vi "Attenuator Initialize Test VNA.vi"(0 "Instrument Record":T10, 5 "Parent VI Refnum":refnum<vi>, 7 "Timing Metrics In":string, 9 "Test Parameters In":T11={"Stimulus"={"ATT Stimulus"={"Normalize"=TRUE, "Value (dB)"=0.0}, "VNA Stimulus"={"Use Instrument Settings"=FALSE, "Blank Frequencies"=FALSE, "Sweep Type"=enum."Linear", "Sweep"={"Fstart"=500.0, "Fstop"=1500.0, "Units"=enum."MHz", "Points"=201}, "Power (dBm)"=999.0, "IFBW (Hz)"=-1.0, "Sweep Time (s)"=-1.0, "Calibration"={"State"=FALSE, "String"=""}}}, "Measurement"={"Step (dB)"=enum."0.25", "Start (dB)"=0.0, "Stop (dB)"=31.75}, "Limit"={"Maximum Error"=0.3}, "Normalization"={"Normalized?"=FALSE, "Normalization Values (dB)"=[]}} {"Stimulus"."VNA Stimulus"."Sweep Time (s)" format="%.3g"}, 11 "error in (no error)":errorcluster, 12 "Miscellaneous Parameters":T1) -> (4 "Instrument ID":string, 6 "Next Action":string, 8 "Timing Metrics Out":string, 10 "Test Parameters Out":T11={"Stimulus"={"ATT Stimulus"={"Normalize"=TRUE, "Value (dB)"=0.0}, "VNA Stimulus"={"Use Instrument Settings"=FALSE, "Blank Frequencies"=FALSE, "Sweep Type"=enum."Linear", "Sweep"={"Fstart"=500.0, "Fstop"=1500.0, "Units"=enum."MHz", "Points"=201}, "Power (dBm)"=999.0, "IFBW (Hz)"=-1.0, "Sweep Time (s)"=-1.0, "Calibration"={"State"=FALSE, "String"=""}}}, "Measurement"={"Step (dB)"=enum."0.25", "Start (dB)"=0.0, "Stop (dB)"=31.75}, "Limit"={"Maximum Error"=0.3}, "Normalization"={"Normalized?"=FALSE, "Normalization Values (dB)"=[]}} {"Stimulus"."VNA Stimulus"."Sweep Time (s)" format="%.3g"}, 14 "Driver Ref":T6, 15 "error out":errorcluster {"code" format="%.0x"})   [LabVIEW 2011]
uses:
  TypeDefs/Attenuator Test Parameters.ctl
  TypeDefs/Attenuator Stimulus Parameters.ctl
  TypeDefs/Attenuator ATT Stimulus.ctl
  TypeDefs/Attenuator VNA Stimulus.ctl
  S Parameter/TypeDefs/SP Frequency Units.ctl
  TypeDefs/Attenuator VNA Calibration State.ctl
  TypeDefs/Attenuator Measurement Cluster.ctl
  TypeDefs/Attenuator Limit.ctl
  TypeDefs/Attenuator Calibration State.ctl
  server/database/Stations/Instruments/Instrument Record.ctl
  TypeDefs/Attenuator Driver Refs.ctl
  drivers/ATT/ATT Driver Ref.ctl
  drivers/VNA/VNA Driver Ref.ctl
  drivers/SNA/SNA Driver Ref.ctl
  TypeDefs/Attenuator Parameter to Measure.ctl
  S Parameter/TypeDefs/SP Parameter.ctl
  S Parameter/TypeDefs/SP Measurement Format.ctl
  S Parameter/TypeDefs/SP Miscellaneous Parameters.ctl
  drivers/VNA/VNA Command.ctl
  drivers/SNA/SNA Command.ctl
panel:
  out "Parameters to Measure":T2[](array[typedef]) {"Channel" min=1 max=99 step=1; "Parameter"."Stimulus Port" min=1 step=1; "Parameter"."Response Port" min=1 step=1}
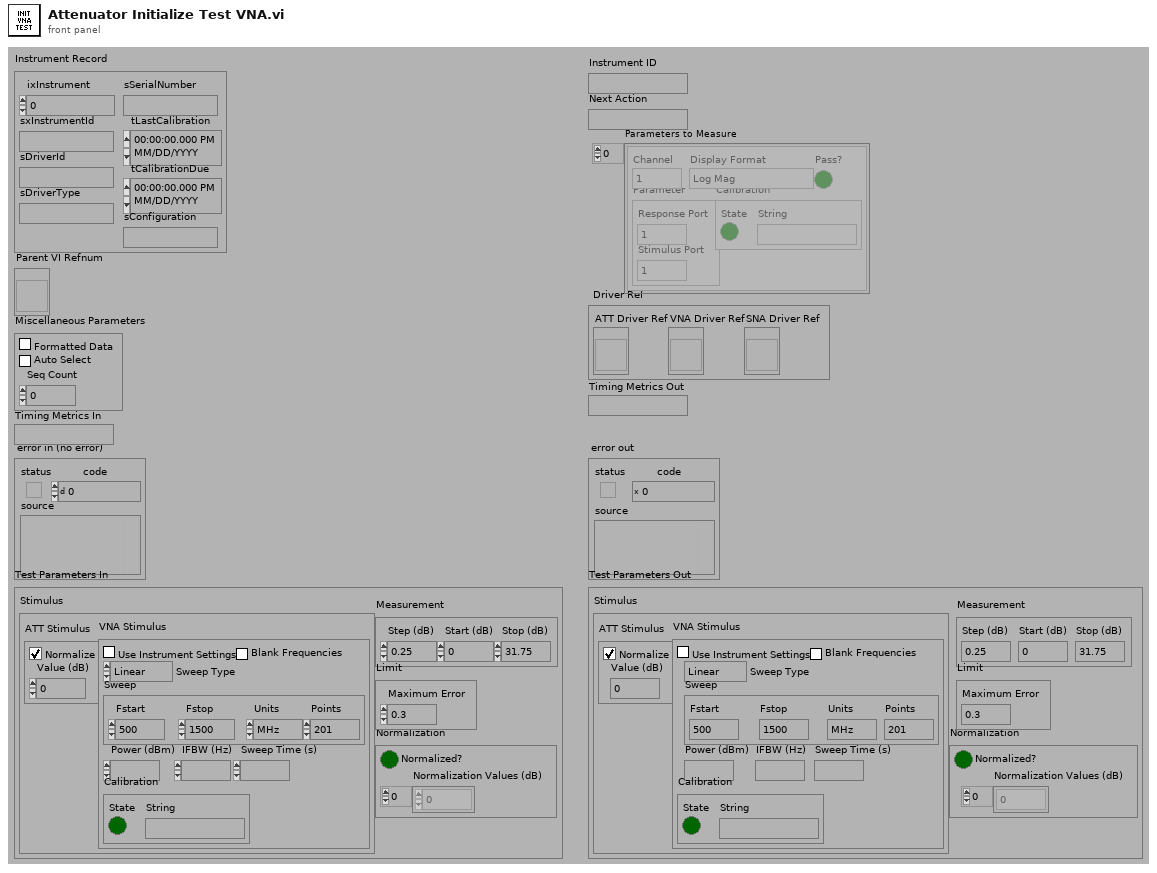
[diagram p1: front panel]
types:
  T1 = typedef "SP Miscellaneous Parameters.ctl" = cluster{"Formatted Data":bool, "Auto Select":bool, "Seq Count":u32}
  T2 = typedef "Attenuator Parameter to Measure.ctl" = cluster{"Channel":i8, "Parameter":T3, "Calibration":T4, "Display Format":T5, "Pass?":bool}
  T3 = typedef "SP Parameter.ctl" = cluster{"Stimulus Port":i8, "Response Port":i8}
  T4 = typedef "Attenuator VNA Calibration State.ctl" = cluster{"State":bool, "String":string}
  T5 = typedef "SP Measurement Format.ctl" = enum32{"Log Mag", "Phase", "Delay", "Smith (R+jX)", "Polar (Re/Im)", "Linear Mag", "SWR", "Real", "Imaginary", "Smith (Lin/Phase)", "Smith (Log/Phase)", "Smith (Real/Imag)", "Smith (G+jB)", "Polar (Lin/Phase)", "Polar (Log/Phase)", "Expanded Phase", "Positive Phase", "Inverted Smith", "Unwrapped Phase", "Power Out", "Power In", "Linear Mag/Phase", "Log Mag/Phase", "Real/Imaginary"}
  T6 = typedef "Attenuator Driver Refs.ctl" = cluster{"ATT Driver Ref":T7, "VNA Driver Ref":T8, "SNA Driver Ref":T9}
  T7 = typedef "ATT Driver Ref.ctl" = refnum<vi>
  T8 = typedef "VNA Driver Ref.ctl" = refnum<vi>
  T9 = typedef "SNA Driver Ref.ctl" = refnum<vi>
  T10 = typedef "Instrument Record.ctl" = cluster{"ixInstrument":i32, "sxInstrumentId":string, "sDriverId":string, "sDriverType":string, "sSerialNumber":string, "tLastCalibration":timestamp, "tCalibrationDue":timestamp, "sConfiguration":string}
  T11 = typedef "Attenuator Test Parameters.ctl" = cluster{"Stimulus":T12, "Measurement":T16, "Limit":T17, "Normalization":T18}
  T12 = typedef "Attenuator Stimulus Parameters.ctl" = cluster{"ATT Stimulus":T13, "VNA Stimulus":T14}
  T13 = typedef "Attenuator ATT Stimulus.ctl" = cluster{"Normalize":bool, "Value (dB)":dbl}
  T14 = typedef "Attenuator VNA Stimulus.ctl" = cluster{"Use Instrument Settings":bool, "Blank Frequencies":bool, "Sweep Type":enum32{"Linear", "Logarithmic", "List", "Power", "CW"}, "Sweep":cluster{"Fstart":dbl, "Fstop":dbl, "Units":T15, "Points":i32}, "Power (dBm)":dbl, "IFBW (Hz)":dbl, "Sweep Time (s)":dbl, "Calibration":T4}
  T15 = typedef "SP Frequency Units.ctl" = enum16{"Hz", "kHz", "MHz", "GHz", "Points"}
  T16 = typedef "Attenuator Measurement Cluster.ctl" = cluster{"Step (dB)":enum16{"0.25", "0.50", "1.00"}, "Start (dB)":dbl, "Stop (dB)":dbl}
  T17 = typedef "Attenuator Limit.ctl" = cluster{"Maximum Error":dbl}
  T18 = typedef "Attenuator Calibration State.ctl" = cluster{"Normalized?":bool, "Normalization Values (dB)":dbl[]}
  T19 = typedef "VNA Command.ctl" = enum16{"LOAD", "INITIALIZE", "PRESET", "GET STIMULUS", "SET STIMULUS", "GET CALIBRATION", "CALIBRATE", "RESTORE", "MEASURE", "RELEASE", "UNLOAD", "CONFIRM", "SORT"}
  T20 = typedef "SNA Command.ctl" = enum16{"LOAD", "INITIALIZE", "PRESET", "GET STIMULUS", "SET STIMULUS", "GET CALIBRATION", "CALIBRATE", "RESTORE", "MEASURE", "RELEASE", "UNLOAD", "CONFIRM", "SORT"}
  T21 = typedef "SP Parameter to Measure.ctl" = cluster{"Channel":i8, "Parameter":T3, "Calibration":T22, "Display Format":T5, "Pass?":bool}
  T22 = typedef "SP Calibration State.ctl" = cluster{"State":bool, "String":string}
  T23 = enum16{"None", "Calibrate", "Restore", "Ignore", "Abort"}
  T24 = typedef "Attenuator Dialog Response.ctl" = enum16{"None", "Calibrate", "Restore", "Ignore", "Abort", "Abort All"}
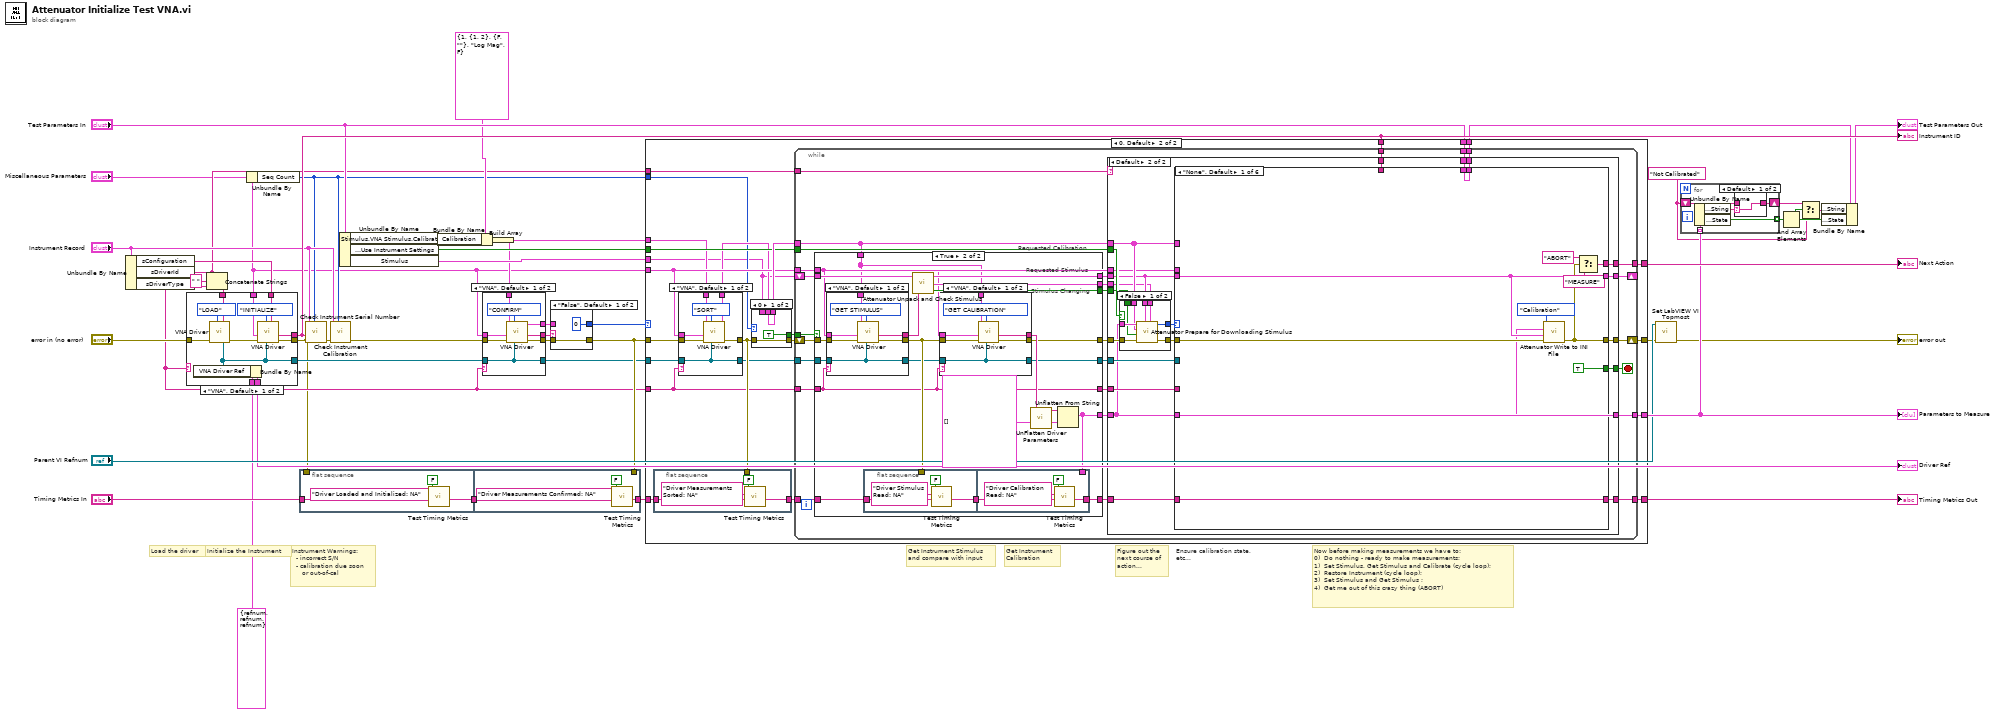
[diagram p0: block diagram]
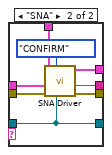
[diagram p3: hidden frame]
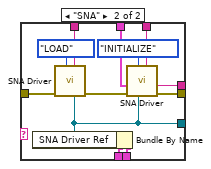
[diagram p4: hidden frame]
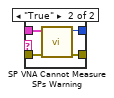
[diagram p5: hidden frame]
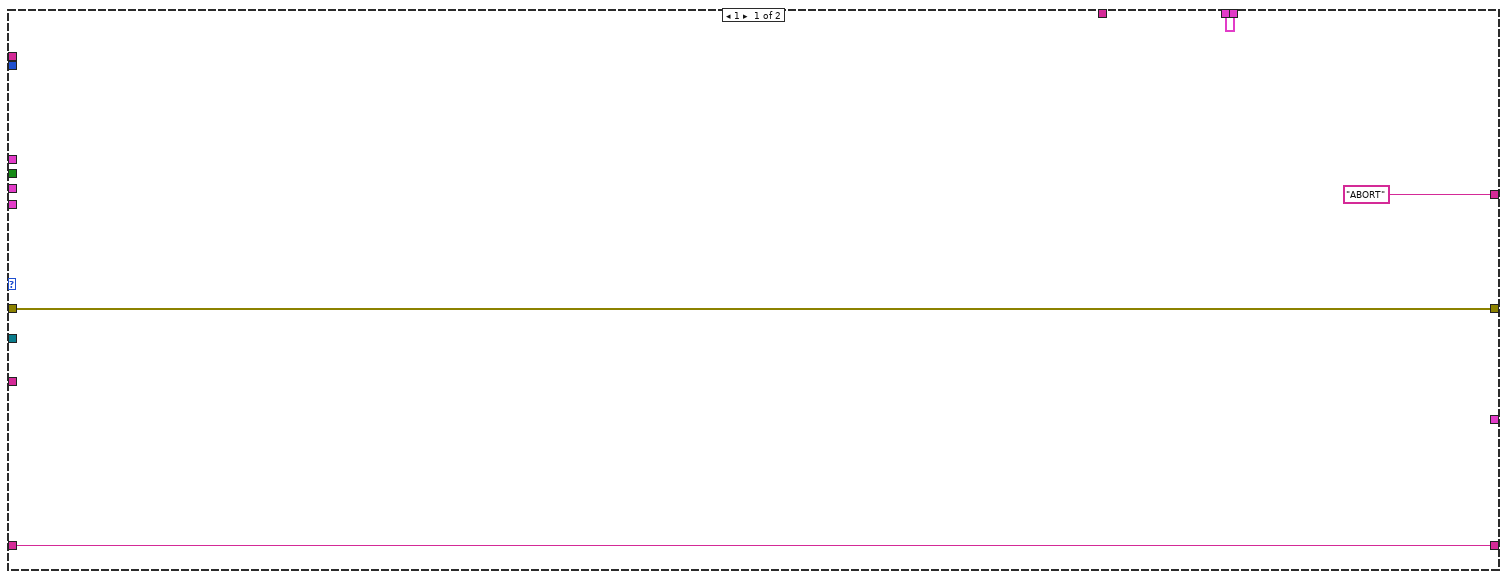
[diagram p6: hidden frame]
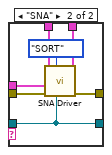
[diagram p7: hidden frame]
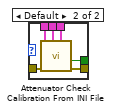
[diagram p8: hidden frame]
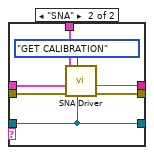
[diagram p10: hidden frame]
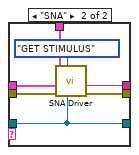
[diagram p11: hidden frame]
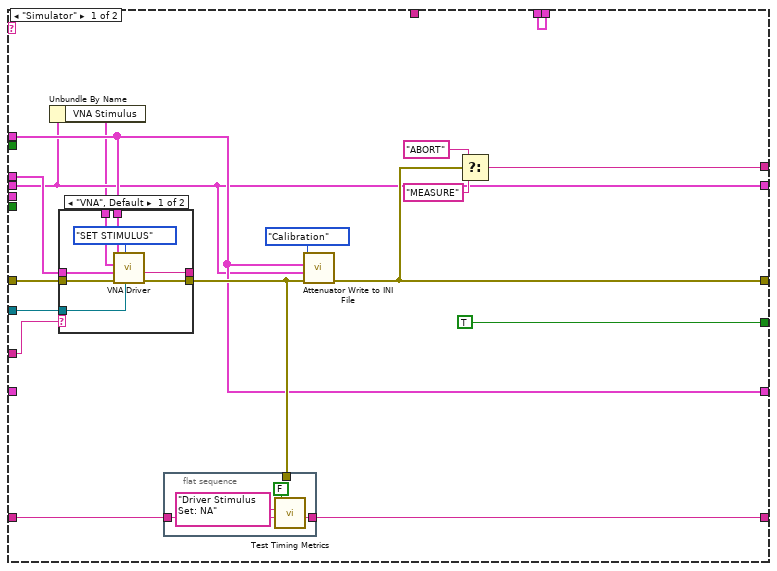
[diagram p12: hidden frame]
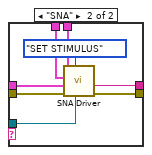
[diagram p13: hidden frame]
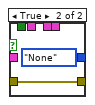
[diagram p14: hidden frame]
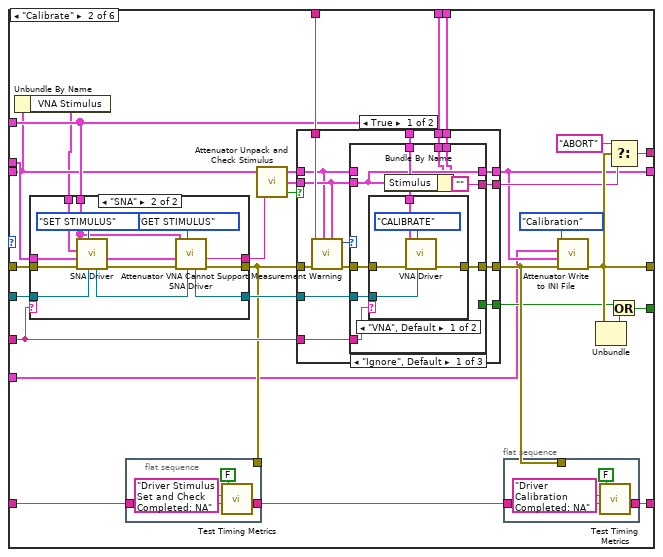
[diagram p15: hidden frame]
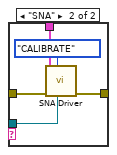
[diagram p16: hidden frame]
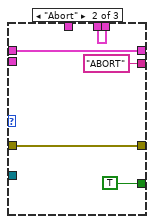
[diagram p17: hidden frame]
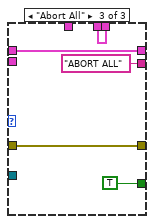
[diagram p18: hidden frame]
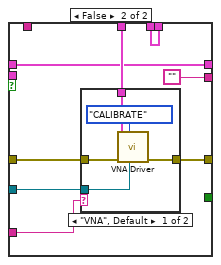
[diagram p19: hidden frame]
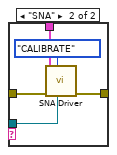
[diagram p20: hidden frame]
diagram:
  w5 = "Not Calibrated"
  # "Now before making measurements we have to:\n0)  Do nothing - ready to make measurements;\n1)  Set Stimulus, Get Stimulus and Calibrate (cycle loop);\n2)  Restore Instrument (cycle loop);\n3)  Set Stimulus and Get Stimulus ;\n4)  Get me out of this crazy thing (ABORT)"
  # "Figure out the\nnext course of\naction..."
  # "Get Instrument\nCalibration"
  # "Instrument Warnings:\n  - incorrect S/N\n  - calibration due soon\n     or out-of-cal"
  # "Get Instrument Stimulus\nand compare with input"
  # "Initialize the Instrument"
  # "Load the driver"
  n1 = Unbundle By Name("Instrument Record") -> ("sConfiguration"=w23:string, "sDriverId"=w22:string, "sDriverType"=w14:string)
  n2 = Concatenate Strings(w22, " " ("string"), w14) -> (w24:string)
  n3 = case shown="\"VNA\", Default" w14 {
    tunnel: "error in (no error)" -> [w55 w67]
    tunnel: [w54 w66] -> w45
    tunnel: w24 -> [w53 w65]
    tunnel: w23 -> [w52 w64]
    tunnel: T6 {"ATT Driver Ref"=refnum, "VNA Driver Ref"=refnum, "SNA Driver Ref"=refnum} ("Driver Ref") -> [w51 w63]
    tunnel: [w50 w62] -> w37
    tunnel: [w48 w58] -> w13
    tunnel: [w47 w60] -> w11
    tunnel: "Miscellaneous Parameters" -> [w46 w59]
    frame "VNA", Default {
      n4 = call "VNA Driver.vi"("VNA Driver or\nVNA Configuration (\"\")"=w53, "VNA Command"=VNA_Command."LOAD", "error in (no error)"=w55) -> ("error out"=w49:errorcluster, "dup Drv Refnum"=w48:T8)  [unwired: 4 in, 3 out]
      n5 = Bundle By Name(cluster=w51, "VNA Driver Ref"=w48) -> (w50:T6)
      n6 = call "VNA Driver.vi"("VNA Driver or\nVNA Configuration (\"\")"=w52, "Drv Refnum"=w48, "VNA Command"=VNA_Command."INITIALIZE", "error in (no error)"=w49, "Miscellaneous Parameters"=w46) -> ("error out"=w47:errorcluster, "VNA Flat Output"=w54:string)  [unwired: 2 in, 3 out]
    }
    frame "SNA" {
      n7 = call "SNA Driver.vi"("SNA Driver or\nSNA Configuration (\"\")"=w65, "SNA Command"=SNA_Command."LOAD", "error in (no error)"=w67) -> ("error out"=w61:errorcluster, "dup Drv Refnum"=w58:T9)  [unwired: 4 in, 3 out]
      n8 = Bundle By Name(cluster=w63, "SNA Driver Ref"=w58) -> (w62:T6)
      n9 = call "SNA Driver.vi"("SNA Driver or\nSNA Configuration (\"\")"=w64, "Drv Refnum"=w58, "SNA Command"=SNA_Command."INITIALIZE", "error in (no error)"=w61, "Miscellaneous Parameters"=w59) -> ("error out"=w60:errorcluster, "SNA Flat Output"=w66:string)  [unwired: 2 in, 3 out]
    }
  }
  "Instrument ID" <- w45
  "Driver Ref" <- w37
  n10 = Unbundle By Name("Miscellaneous Parameters") -> ("Seq Count"=w2:u32)
  n11 = flat-sequence {
    tunnel: [w71] -> w33
    tunnel: w11 -> [_]
    tunnel: "Timing Metrics In" -> [w70]
    tunnel: w33 -> [w75]
    tunnel: w16 -> [_]
    tunnel: [w74] -> w15
    frame #0 {
      n12 = call "Test Timing Metrics.vi"("Start?"=FALSE, "Timing Metrics In"=w70, "Message"="Driver Loaded and Initialized: NA") -> ("Timing Metrics Out"=w71:string)  [unwired: 6 out]
    }
    frame #1 {
      n13 = call "Test Timing Metrics.vi"("Start?"=FALSE, "Timing Metrics In"=w75, "Message"="Driver Measurements Confirmed: NA") -> ("Timing Metrics Out"=w74:string)  [unwired: 6 out]
    }
  }
  n14 = call "Check Instrument Serial Number.vi"("Seq Count"=w2, "error in (no error)"=w11, "Instrument IDN String (\"\")"=w45, "Instrument Record"="Instrument Record") -> ("error out"=w31:errorcluster)  [unwired: 7 out]
  n15 = call "Check Instrument Calibration.vi"("Seq Count"=w2, "error in (no error)"=w31, "Instrument Record"="Instrument Record") -> ("error out"=w21:errorcluster)  [unwired: 8 out]
  n16 = Unbundle By Name("Test Parameters In") -> ("Stimulus.VNA Stimulus.Calibration"=w28:T4, "Stimulus.VNA Stimulus.Use Instrument Settings"=w26:bool, "Stimulus"=w27:T12)
  n17 = Bundle By Name(cluster=T2 {"Channel"=1, "Parameter"={"Stimulus Port"=1, "Response Port"=2}, "Calibration"={"State"=FALSE, "String"=""}, "Display Format"=enum."Log Mag", "Pass?"=FALSE} ("Parameter to Measure"), "Calibration"=w28) -> (w4:T2)
  n18 = Build Array(w4) -> (w3:T2[])
  n19 = case shown="\"VNA\", Default" w14 {
    tunnel: w21 -> [w84 w92]
    tunnel: "Miscellaneous Parameters" -> [w83 w91]
    tunnel: [w82 w90] -> w20
    tunnel: [w81 w89] -> w19
    tunnel: w3 -> [w80 w88]
    tunnel: [w79 w87] -> w17
    tunnel: w13 -> [w78 w86]
    tunnel: [w78 w86] -> w12
    frame "VNA", Default {
      n20 = call "VNA Driver.vi"("Drv Refnum"=w78, "VNA Command"=VNA_Command."CONFIRM", "error in (no error)"=w84, "Miscellaneous Parameters"=w83, "Parameters to Measure"=w80) -> ("error out"=w79:errorcluster, "VNA Flat Output"=w82:string, "Parameters Measured"=w81:T21[])  [unwired: 2 in, 2 out]
    }
    frame "SNA" {
      n21 = call "SNA Driver.vi"("Drv Refnum"=w86, "SNA Command"=SNA_Command."CONFIRM", "error in (no error)"=w92, "Miscellaneous Parameters"=w91, "Parameters to Measure"=w88) -> ("error out"=w87:errorcluster, "SNA Flat Output"=w90:string, "Parameters Measured"=w89:T21[])  [unwired: 2 in, 2 out]
    }
  }
  n22 = case shown="\"False\", Default" w20 {
    tunnel: w17 -> [w95 w99]
    tunnel: [w95 w98] -> w16
    tunnel: w19 -> [_ w97]
    tunnel: [0 ("Choice") w96] -> w18
    frame "False", Default {
    }
    frame "True" {
      n23 = call "SP VNA Cannot Measure SPs Warning.vi"("error in (no error)"=w99, "Removed Parameters"=w97) -> ("error out"=w98:errorcluster, "Choice"=w96:i32)  [unwired: 8 out]
    }
  }
  n24 = case shown="0, Default" w18 {
    tunnel: ["ABORT" w127] -> w43
    tunnel: [_ w124] -> w42
    tunnel: [w103 w123] -> w30
    tunnel: w27 -> [_ w104]
    tunnel: w26 -> [_ w121]
    tunnel: w22 -> [_ w120]
    tunnel: w16 -> [w103 w115]
    tunnel: "Miscellaneous Parameters" -> [_ w114]
    tunnel: w3 -> [_ w113]
    tunnel: w15 -> [w101 w119]
    tunnel: [w101 w117] -> w35
    tunnel: w14 -> [_ w109]
    tunnel: w12 -> [_ w111]
    tunnel: w45 -> [_ w108]
    tunnel: "Test Parameters In" -> [w100 w107]
    tunnel: [w100 w106] -> w9
    tunnel: w2 -> [_ w105]
    frame 1 {
    }
    frame 0, Default {
      n25 = flat-sequence {
        tunnel: w119 -> [w143]
        tunnel: [w142] -> w118
        tunnel: w116 -> [_]
        frame #0 {
          n26 = call "Test Timing Metrics.vi"("Start?"=FALSE, "Timing Metrics In"=w143, "Message"="Driver Measurements Sorted: NA") -> ("Timing Metrics Out"=w142:string)  [unwired: 6 out]
        }
      }
      n27 = case shown="\"VNA\", Default" w109 {
        tunnel: w115 -> [w133 w140]
        tunnel: w114 -> [w132 w139]
        tunnel: w113 -> [w131 w138]
        tunnel: [w130 w137] -> w116
        tunnel: [w129 w136] -> w112
        tunnel: w111 -> [w128 w135]
        tunnel: [w128 w135] -> w110
        frame "VNA", Default {
          n28 = call "VNA Driver.vi"("Drv Refnum"=w128, "VNA Command"=VNA_Command."SORT", "error in (no error)"=w133, "Miscellaneous Parameters"=w132, "Parameters to Measure"=w131) -> ("error out"=w130:errorcluster, "Parameters Measured"=w129:T21[])  [unwired: 2 in, 3 out]
        }
        frame "SNA" {
          n29 = call "SNA Driver.vi"("Drv Refnum"=w135, "SNA Command"=SNA_Command."SORT", "error in (no error)"=w140, "Miscellaneous Parameters"=w139, "Parameters to Measure"=w138) -> ("error out"=w137:errorcluster, "Parameters Measured"=w136:T21[])  [unwired: 2 in, 3 out]
        }
      }
      n30 = case shown="0" w105 {
        tunnel: w116 -> [w148 w154]
        tunnel: [w148 w153] -> w126
        tunnel: [TRUE ("Check Instrument") w152] -> w125
        tunnel: w112 -> [w146 w151]
        tunnel: w104 -> [_ w150]
        tunnel: [w146 w149] -> w122
        frame 0 {
        }
        frame Default {
          n31 = call "Attenuator Check Calibration From INI File.vi"("Paramters to Measure"=w151, "error in (no error)"=w154, "Requested Stimulus"=w150) -> ("error out"=w153:errorcluster, "Check Instrument"=w152:bool, "Paramters to Measure Out"=w149:T2[])  [unwired: 5 in, 1 out]
        }
      }
      n32 = while "Ensure calibration state, etc..." {
        shift-right: [w180] -> w123
        shift-left: w126 -> [w169]
        tunnel: [w179] -> w127
        tunnel: [w177] -> w124
        tunnel: w120 -> [w176]
        tunnel: w122 -> [w155]
        tunnel: w125 -> [w170]
        tunnel: w121 -> [w168]
        tunnel: w114 -> [w166]
        tunnel: w118 -> [w165]
        tunnel: [w163] -> w117
        tunnel: w110 -> [w162]
        tunnel: w109 -> [w161]
        tunnel: w108 -> [w159]
        tunnel: w107 -> [w158]
        tunnel: [w157] -> w106
        shift-right: [w156] -> _
        shift-left: w104 -> [w171]
        stop <- w181 stop-if-true
        # "Requested Calibration"
        n33 = case shown="True" w170 {
          selector: w170 -> [w187 _]
          tunnel: [w182 w202] -> w178
          tunnel: [w188 w196] -> w175
          tunnel: [w187 w207] -> w174
          tunnel: [w186 w208] -> w173
          tunnel: w169 -> [w188 w200]
          tunnel: w171 -> [w186 w206]
          tunnel: [w184 w192] -> w172
          tunnel: [w186 w205] -> w167
          tunnel: w155 -> [w182 w191]
          tunnel: w166 -> [_ w195]
          tunnel: w165 -> [w185 w204]
          tunnel: [w185 w201] -> w164
          tunnel: w162 -> [w184 w199]
          tunnel: w161 -> [w183 w190]
          tunnel: [w183 w190] -> w160
          frame False {
            # "Don't check instrument.\nSettings are the same as last run.\nSave time."
          }
          frame True {
            # "Requested Stimulus"
            # "Stimulus Changing"
            n34 = case shown="\"VNA\", Default" w190 {
              tunnel: w200 -> [w230 w237]
              tunnel: w195 -> [w229 w236]
              tunnel: w191 -> [w228 w235]
              tunnel: [w227 w234] -> w194
              tunnel: w199 -> [w226 w233]
              tunnel: [w226 w233] -> w193
              tunnel: [w225 w232] -> w198
              frame "VNA", Default {
                n35 = call "VNA Driver.vi"("Drv Refnum"=w226, "VNA Command"=VNA_Command."GET STIMULUS", "error in (no error)"=w230, "Miscellaneous Parameters"=w229, "Parameters to Measure"=w228) -> ("error out"=w227:errorcluster, "VNA Flat Output"=w225:string)  [unwired: 2 in, 3 out]
              }
              frame "SNA" {
                n36 = call "SNA Driver.vi"("Drv Refnum"=w233, "SNA Command"=SNA_Command."GET STIMULUS", "error in (no error)"=w237, "Miscellaneous Parameters"=w236, "Parameters to Measure"=w235) -> ("error out"=w234:errorcluster, "SNA Flat Output"=w232:string)  [unwired: 2 in, 3 out]
              }
            }
            n37 = flat-sequence {
              tunnel: w204 -> [w239]
              tunnel: w194 -> [_]
              tunnel: [w238] -> w203
              tunnel: w203 -> [w243]
              tunnel: w202 -> [_]
              tunnel: [w242] -> w201
              frame #0 {
                n38 = call "Test Timing Metrics.vi"("Start?"=FALSE, "Timing Metrics In"=w239, "Message"="Driver Stimulus Read: NA") -> ("Timing Metrics Out"=w238:string)  [unwired: 6 out]
              }
              frame #1 {
                n39 = call "Test Timing Metrics.vi"("Start?"=FALSE, "Timing Metrics In"=w243, "Message"="Driver Calibration Read: NA") -> ("Timing Metrics Out"=w242:string)  [unwired: 6 out]
              }
            }
            n40 = call "Attenuator Unpack and Check Stimulus.vi"("Flat Stimulus"=w198, "Requested Stimulus In"=w206) -> ("Stimulus Changed?"=w207:bool, "Current Stimulus"=w205:T12, "Requested Stimulus Out"=w208:T12)  [unwired: 1 out]
            n41 = case shown="\"VNA\", Default" w190 {
              tunnel: w194 -> [w216 w223]
              tunnel: w195 -> [w215 w222]
              tunnel: w191 -> [w214 w221]
              tunnel: [w213 w220] -> w196
              tunnel: w193 -> [w212 w219]
              tunnel: [w212 w219] -> w192
              tunnel: [w211 w218] -> w197
              frame "VNA", Default {
                n42 = call "VNA Driver.vi"("Drv Refnum"=w212, "VNA Command"=VNA_Command."GET CALIBRATION", "error in (no error)"=w216, "Miscellaneous Parameters"=w215, "Parameters to Measure"=w214) -> ("error out"=w213:errorcluster, "VNA Flat Output"=w211:string)  [unwired: 2 in, 3 out]
              }
              frame "SNA" {
                n43 = call "SNA Driver.vi"("Drv Refnum"=w219, "SNA Command"=SNA_Command."GET CALIBRATION", "error in (no error)"=w223, "Miscellaneous Parameters"=w222, "Parameters to Measure"=w221) -> ("error out"=w220:errorcluster, "SNA Flat Output"=w218:string)  [unwired: 2 in, 3 out]
              }
            }
            n44 = call "UnFlatten Driver Parameters.vi"("Flattened Driver Parameters with Version (\"\")"=w197) -> ("Flat Driver Parameters"=w209:string)  [unwired: 1 in, 5 out]
            n45 = Unflatten From String(type=T2[] [] ("Parameters Measured"), binary string=w209) -> (value=w202:T2[])  [unwired: 1 in, 4 out]
          }
        }
        n46 = case shown="Default" w176 {
          tunnel: [TRUE w303] -> w181
          tunnel: [w258 w302] -> w180
          tunnel: [w260 w301] -> w179
          tunnel: w173 -> [w247 w294]
          tunnel: w172 -> [w251 w300]
          tunnel: w178 -> [_ w283]
          tunnel: [w248 w283] -> w177
          tunnel: w175 -> [w253 w299]
          tunnel: w155 -> [w248 w296]
          tunnel: w174 -> [_ w288]
          tunnel: w168 -> [_ w295]
          tunnel: w167 -> [_ w293]
          tunnel: w166 -> [w254 w292]
          tunnel: w164 -> [w255 w291]
          tunnel: [w256 w290] -> w163
          tunnel: w160 -> [w250 w289]
          tunnel: w159 -> [_ w287]
          tunnel: w158 -> [w249 w286]
          tunnel: [w249 w285] -> w157
          tunnel: [w247 w284] -> w156
          frame "Simulator" {
            n47 = Unbundle By Name(w247) -> ("VNA Stimulus"=w246:T14)
            n48 = case shown="\"VNA\", Default" w250 {
              tunnel: w253 -> [w270 w278]
              tunnel: w254 -> [w269 w277]
              tunnel: w248 -> [w268 w276]
              tunnel: [w267 w275] -> w252
              tunnel: w251 -> [w266 w274]
              tunnel: [w265 w273] -> _
              tunnel: w246 -> [w263 w271]
              frame "VNA", Default {
                n49 = call "VNA Driver.vi"("Drv Refnum"=w266, "VNA Command"=VNA_Command."SET STIMULUS", "error in (no error)"=w270, "Miscellaneous Parameters"=w269, "VNA Stimulus"=w263, "Parameters to Measure"=w268) -> ("error out"=w267:errorcluster, "VNA Flat Output"=w265:string)  [unwired: 1 in, 3 out]
              }
              frame "SNA" {
                n50 = call "SNA Driver.vi"("Drv Refnum"=w274, "SNA Command"=SNA_Command."SET STIMULUS", "error in (no error)"=w278, "Miscellaneous Parameters"=w277, "SNA Stimulus"=w271, "Parameters to Measure"=w276) -> ("error out"=w275:errorcluster, "SNA Flat Output"=w273:string)  [unwired: 1 in, 3 out]
              }
            }
            n51 = flat-sequence {
              tunnel: [w279] -> w256
              tunnel: w255 -> [w280]
              tunnel: w252 -> [_]
              frame #0 {
                n52 = call "Test Timing Metrics.vi"("Start?"=FALSE, "Timing Metrics In"=w280, "Message"="Driver Stimulus Set: NA") -> ("Timing Metrics Out"=w279:string)  [unwired: 6 out]
              }
            }
            n53 = call "Attenuator Write to INI File.vi"("error in (no error)"=w252, "Requested Stimulus"=w247, "Parameters to Measure"=w248, "Data to Write"=enum16{"Calibration", "Display", "De-Embed"}."Calibration") -> ("error out"=w258:errorcluster)  [unwired: 2 in, 5 out]
            n54 = Select(t="ABORT", s=w258, f="MEASURE") -> (s? t:f=w260:string)
          }
          frame Default {
            n55 = case shown="False" w295 {
              tunnel: w299 -> [w311 w313]
              tunnel: [w310 w313] -> w298
              tunnel: [w309 T23."None" ("Action")] -> w297
              tunnel: w283 -> [w308 _]
              tunnel: w288 -> [w307 _]
              tunnel: w296 -> [w306 _]
              tunnel: w294 -> [w305 _]
              tunnel: w293 -> [w304 _]
              frame False {
                n56 = call "Attenuator Prepare for Downloading Stimulus.vi"("Current Stimulus"=w304, "Requested Stimulus"=w305, "error in (no error)"=w311, "Stimulus Changing? (f)"=w307, "Parameters to Measure"=w306, "Currnet Parameters to Measure"=w308) -> ("error out"=w310:errorcluster, "Action"=w309:T24)  [unwired: 1 in, 3 out]
              }
              frame True {
              }
            }
            n57 = case shown="\"None\", Default" w297 {
              tunnel: w298 -> [w320 w349 w456 w490 w569 w577]
              tunnel: [w319 w352 w460 w501 w568 w576] -> w302
              tunnel: [TRUE w334 w461 TRUE TRUE TRUE] -> w303
              tunnel: [w322 w353 w462 w505 "ABORT" "ABORT ALL"] -> w301
              tunnel: w300 -> [_ w348 w454 w498 _ _]
              tunnel: w296 -> [_ w327 w449 w481 _ _]
              tunnel: w294 -> [w315 w326 w451 w480 w565 w573]
              tunnel: w292 -> [_ w347 _ w489 _ _]
              tunnel: w291 -> [w317 w342 w458 w497 w567 w575]
              tunnel: [w317 w350 w457 w496 w567 w575] -> w290
              tunnel: w289 -> [_ w344 w453 w491 _ _]
              tunnel: w287 -> [_ w339 _ w487 _ _]
              tunnel: w286 -> [w316 w331 w452 w485 w566 w574]
              tunnel: [w316 w330 w452 w484 w566 w574] -> w285
              tunnel: [w315 w329 w451 w483 w565 w573] -> w284
              tunnel: w283 -> [w314 w328 w450 w482 w564 w572]
              frame "None", Default {
                n58 = call "Attenuator Write to INI File.vi"("error in (no error)"=w320, "Requested Stimulus"=w315, "Parameters to Measure"=w314, "Data to Write"=enum16{"Calibration", "Display", "De-Embed"}."Calibration") -> ("error out"=w319:errorcluster)  [unwired: 2 in, 5 out]
                n59 = Select(t="ABORT", s=w319, f="MEASURE") -> (s? t:f=w322:string)
              }
              frame "Calibrate" {
                n60 = Unbundle By Name(w326) -> ("VNA Stimulus"=w325:T14)
                n61 = case shown="\"SNA\"" w344 {
                  tunnel: w349 -> [w432 w444]
                  tunnel: w347 -> [w431 w435]
                  tunnel: w327 -> [w424 w439]
                  tunnel: [w427 w440] -> w340
                  tunnel: w348 -> [w429 w438]
                  tunnel: [w423 w436] -> w345
                  tunnel: [w422 w434] -> w343
                  tunnel: w325 -> [w421 w433]
                  frame "VNA", Default {
                    n62 = call "VNA Driver.vi"("Drv Refnum"=w429, "VNA Command"=VNA_Command."SET STIMULUS", "error in (no error)"=w432, "Miscellaneous Parameters"=w431, "VNA Stimulus"=w421, "Parameters to Measure"=w424) -> ("error out"=w425:errorcluster, "dup Drv Refnum"=w428:T8)  [unwired: 1 in, 3 out]
                    n63 = call "VNA Driver.vi"("Drv Refnum"=w428, "VNA Command"=VNA_Command."GET STIMULUS", "error in (no error)"=w425, "Parameters to Measure"=w424) -> ("error out"=w427:errorcluster, "VNA Flat Output"=w422:string, "dup Drv Refnum"=w423:T8)  [unwired: 3 in, 2 out]
                  }
                  frame "SNA" {
                    n64 = call "SNA Driver.vi"("Drv Refnum"=w438, "SNA Command"=SNA_Command."SET STIMULUS", "error in (no error)"=w444, "Miscellaneous Parameters"=w435, "SNA Stimulus"=w433, "Parameters to Measure"=w439) -> ("error out"=w441:errorcluster, "dup Drv Refnum"=w437:T9)  [unwired: 1 in, 3 out]
                    n65 = call "SNA Driver.vi"("Drv Refnum"=w437, "SNA Command"=SNA_Command."GET STIMULUS", "error in (no error)"=w441, "Miscellaneous Parameters"=w435, "Parameters to Measure"=w439) -> ("error out"=w440:errorcluster, "SNA Flat Output"=w434:string, "dup Drv Refnum"=w436:T9)  [unwired: 2 in, 2 out]
                  }
                }
                n66 = flat-sequence {
                  tunnel: [w418] -> w341
                  tunnel: w342 -> [w417]
                  tunnel: w340 -> [_]
                  frame #0 {
                    n67 = call "Test Timing Metrics.vi"("Start?"=FALSE, "Timing Metrics In"=w417, "Message"="Driver Stimulus Set and Check Completed: NA") -> ("Timing Metrics Out"=w418:string)  [unwired: 6 out]
                  }
                }
                n68 = call "Attenuator Unpack and Check Stimulus.vi"("Flat Stimulus"=w343, "Requested Stimulus In"=w326) -> ("Stimulus Changed?"=w338:bool, "Current Stimulus"=w337:T12, "Requested Stimulus Out"=w336:T12)  [unwired: 1 out]
                n69 = case shown="True" w338 {
                  tunnel: [w369 w406] -> w346
                  tunnel: w345 -> [w368 w405]
                  tunnel: w327 -> [w367 w404]
                  tunnel: w344 -> [w366 w403]
                  tunnel: w340 -> [w364 w401]
                  tunnel: w339 -> [w363 _]
                  tunnel: w337 -> [w361 _]
                  tunnel: w336 -> [w360 w400]
                  tunnel: [w359 w400] -> w329
                  tunnel: [w358 ""] -> w335
                  tunnel: [w357 _] -> w332
                  tunnel: w331 -> [w356 w399]
                  tunnel: [w355 w399] -> w330
                  frame True {
                    n70 = call "Attenuator VNA Cannot Support Measurement Warning.vi"("Current Stimulus"=w361, "Requested Stimulus"=w360, "error in (no error)"=w364, "Instrument IDN String (\"\")"=w363) -> ("error out"=w365:errorcluster, "Choice"=w362:T24)  [unwired: 2 in, 4 out]
                    n71 = case shown="\"Ignore\", Default" w362 {
                      tunnel: [w378 w391 w396] -> w369
                      tunnel: w368 -> [w377 _ _]
                      tunnel: w367 -> [w376 _ _]
                      tunnel: w366 -> [w375 _ _]
                      tunnel: w365 -> [w374 w391 w396]
                      tunnel: w361 -> [w372 _ _]
                      tunnel: w360 -> [_ w393 w398]
                      tunnel: [w372 w393 w398] -> w359
                      tunnel: ["" "ABORT" "ABORT ALL"] -> w358
                      tunnel: [_ TRUE TRUE] -> w357
                      tunnel: w356 -> [w371 w389 w394]
                      tunnel: [w370 w389 w394] -> w355
                      frame "Ignore", Default {
                        n72 = case shown="\"VNA\", Default" w375 {
                          tunnel: w374 -> [w383 w388]
                          tunnel: w376 -> [w380 w386]
                          tunnel: [w379 w384] -> w378
                          tunnel: w377 -> [w381 w385]
                          frame "VNA", Default {
                            n73 = call "VNA Driver.vi"("Drv Refnum"=w381, "VNA Command"=VNA_Command."CALIBRATE", "error in (no error)"=w383, "Parameters to Measure"=w380) -> ("error out"=w379:errorcluster)  [unwired: 3 in, 4 out]
                          }
                          frame "SNA" {
                            n74 = call "SNA Driver.vi"("Drv Refnum"=w385, "SNA Command"=SNA_Command."CALIBRATE", "error in (no error)"=w388, "Parameters to Measure"=w386) -> ("error out"=w384:errorcluster)  [unwired: 3 in, 4 out]
                          }
                        }
                        n75 = Bundle By Name(cluster=w371, "Stimulus"=w372) -> (w370:T11)
                      }
                      frame "Abort" {
                      }
                      frame "Abort All" {
                      }
                    }
                  }
                  frame False {
                    n76 = case shown="\"VNA\", Default" w403 {
                      tunnel: w401 -> [w411 w416]
                      tunnel: w404 -> [w408 w414]
                      tunnel: [w407 w412] -> w406
                      tunnel: w405 -> [w409 w413]
                      frame "VNA", Default {
                        n77 = call "VNA Driver.vi"("Drv Refnum"=w409, "VNA Command"=VNA_Command."CALIBRATE", "error in (no error)"=w411, "Parameters to Measure"=w408) -> ("error out"=w407:errorcluster)  [unwired: 3 in, 4 out]
                      }
                      frame "SNA" {
                        n78 = call "SNA Driver.vi"("Drv Refnum"=w413, "SNA Command"=SNA_Command."CALIBRATE", "error in (no error)"=w416, "Parameters to Measure"=w414) -> ("error out"=w412:errorcluster)  [unwired: 3 in, 4 out]
                      }
                    }
                  }
                }
                n79 = flat-sequence {
                  tunnel: [w446] -> w350
                  tunnel: w341 -> [w445]
                  tunnel: w346 -> [_]
                  frame #0 {
                    n80 = call "Test Timing Metrics.vi"("Start?"=FALSE, "Timing Metrics In"=w445, "Message"="Driver Calibration Completed: NA") -> ("Timing Metrics Out"=w446:string)  [unwired: 6 out]
                  }
                }
                n81 = call "Attenuator Write to INI File.vi"("error in (no error)"=w346, "Requested Stimulus"=w329, "Parameters to Measure"=w328, "Data to Write"=enum16{"Calibration", "Display"}."Calibration") -> ("error out"=w352:errorcluster)  [unwired: 2 in, 5 out]
                n82 = Unbundle(w352) -> ("status"=w333:bool)  [unwired: 2 out]
                n83 = Select(t="ABORT", s=w352, f=w335) -> (s? t:f=w353:string)
                n84 = Or(x=w332, y=w333) -> (x .or. y?=w334:bool)
              }
              frame "Restore" {
                n85 = case shown="\"SNA\"" w453 {
                  tunnel: w456 -> [w469 w474]
                  tunnel: w449 -> [w468 w473]
                  tunnel: [w467 w472] -> w455
                  tunnel: w454 -> [w466 w471]
                  frame "VNA", Default {
                    n86 = call "VNA Driver.vi"("Drv Refnum"=w466, "VNA Command"=VNA_Command."RESTORE", "error in (no error)"=w469, "Parameters to Measure"=w468) -> ("error out"=w467:errorcluster)  [unwired: 3 in, 4 out]
                  }
                  frame "SNA" {
                    n87 = call "SNA Driver.vi"("Drv Refnum"=w471, "SNA Command"=SNA_Command."RESTORE", "error in (no error)"=w474, "Parameters to Measure"=w473) -> ("error out"=w472:errorcluster)  [unwired: 3 in, 4 out]
                  }
                }
                n88 = flat-sequence {
                  tunnel: w458 -> [w476]
                  tunnel: w455 -> [_]
                  tunnel: [w475] -> w457
                  frame #0 {
                    n89 = call "Test Timing Metrics.vi"("Start?"=FALSE, "Timing Metrics In"=w476, "Message"="Driver Calibration Restored: NA") -> ("Timing Metrics Out"=w475:string)  [unwired: 6 out]
                  }
                }
                n90 = call "Attenuator Write to INI File.vi"("error in (no error)"=w455, "Requested Stimulus"=w451, "Parameters to Measure"=w450, "Data to Write"=enum16{"Calibration", "Display", "De-Embed"}."Calibration") -> ("error out"=w460:errorcluster)  [unwired: 2 in, 5 out]
                n91 = Unbundle(w460) -> ("status"=w461:bool)  [unwired: 2 out]
                n92 = Select(t="ABORT", s=w460, f="") -> (s? t:f=w462:string)
              }
              frame "Ignore" {
                n93 = Unbundle By Name(w480) -> ("VNA Stimulus"=w479:T14)
                n94 = case shown="\"SNA\"" w491 {
                  tunnel: w490 -> [w551 w563]
                  tunnel: w489 -> [w550 w554]
                  tunnel: w481 -> [w543 w558]
                  tunnel: [w546 w559] -> w499
                  tunnel: w498 -> [w548 w557]
                  tunnel: [w542 w555] -> w488
                  tunnel: [w541 w553] -> w500
                  tunnel: w479 -> [w540 w552]
                  frame "VNA", Default {
                    n95 = call "VNA Driver.vi"("Drv Refnum"=w548, "VNA Command"=VNA_Command."SET STIMULUS", "error in (no error)"=w551, "Miscellaneous Parameters"=w550, "VNA Stimulus"=w540, "Parameters to Measure"=w543) -> ("error out"=w544:errorcluster, "dup Drv Refnum"=w547:T8)  [unwired: 1 in, 3 out]
                    n96 = call "VNA Driver.vi"("Drv Refnum"=w547, "VNA Command"=VNA_Command."GET STIMULUS", "error in (no error)"=w544, "Parameters to Measure"=w543) -> ("error out"=w546:errorcluster, "VNA Flat Output"=w541:string, "dup Drv Refnum"=w542:T8)  [unwired: 3 in, 2 out]
                  }
                  frame "SNA" {
                    n97 = call "SNA Driver.vi"("Drv Refnum"=w557, "SNA Command"=SNA_Command."SET STIMULUS", "error in (no error)"=w563, "Miscellaneous Parameters"=w554, "SNA Stimulus"=w552, "Parameters to Measure"=w558) -> ("error out"=w560:errorcluster, "dup Drv Refnum"=w556:T9)  [unwired: 1 in, 3 out]
                    n98 = call "SNA Driver.vi"("Drv Refnum"=w556, "SNA Command"=SNA_Command."GET STIMULUS", "error in (no error)"=w560, "Miscellaneous Parameters"=w554, "Parameters to Measure"=w558) -> ("error out"=w559:errorcluster, "SNA Flat Output"=w553:string, "dup Drv Refnum"=w555:T9)  [unwired: 2 in, 2 out]
                  }
                }
                n99 = flat-sequence {
                  tunnel: [w537] -> w496
                  tunnel: w497 -> [w536]
                  tunnel: w499 -> [_]
                  frame #0 {
                    n100 = call "Test Timing Metrics.vi"("Start?"=FALSE, "Timing Metrics In"=w536, "Message"="Driver Stimulus Set and Check Completed: NA") -> ("Timing Metrics Out"=w537:string)  [unwired: 6 out]
                  }
                }
                n101 = call "Attenuator Unpack and Check Stimulus.vi"("Flat Stimulus"=w500, "Requested Stimulus In"=w480) -> ("Stimulus Changed?"=w494:bool, "Current Stimulus"=w493:T12, "Requested Stimulus Out"=w492:T12)  [unwired: 1 out]
                n102 = case shown="False" w494 {
                  tunnel: [w518 w534] -> w495
                  tunnel: w488 -> [w517 _]
                  tunnel: w491 -> [w516 _]
                  tunnel: w499 -> [w514 w534]
                  tunnel: w487 -> [w513 _]
                  tunnel: w493 -> [w511 _]
                  tunnel: w492 -> [w510 w535]
                  tunnel: [w509 w535] -> w483
                  tunnel: [w508 "MEASURE"] -> w486
                  tunnel: w485 -> [w507 w532]
                  tunnel: [w506 w532] -> w484
                  frame True {
                    n103 = call "Attenuator VNA Cannot Support Measurement Warning.vi"("Current Stimulus"=w511, "Requested Stimulus"=w510, "error in (no error)"=w514, "Instrument IDN String (\"\")"=w513) -> ("error out"=w515:errorcluster, "Choice"=w512:T24)  [unwired: 2 in, 4 out]
                    n104 = case shown="\"Abort\"" w512 {
                      tunnel: [w523 w525 w529] -> w518
                      tunnel: w517 -> [_ _ _]
                      tunnel: w516 -> [_ _ _]
                      tunnel: w515 -> [w523 w525 w529]
                      tunnel: w511 -> [w520 _ _]
                      tunnel: w510 -> [_ w527 w531]
                      tunnel: [w520 w527 w531] -> w509
                      tunnel: ["MEASURE" "ABORT" "ABORT ALL"] -> w508
                      tunnel: w507 -> [w521 w524 w528]
                      tunnel: [w519 w524 w528] -> w506
                      frame "Ignore", Default {
                        n105 = Bundle By Name(cluster=w521, "Stimulus"=w520) -> (w519:T11)
                      }
                      frame "Abort" {
                      }
                      frame "Abort All" {
                      }
                    }
                  }
                  frame False {
                  }
                }
                n106 = call "Attenuator Write to INI File.vi"("error in (no error)"=w495, "Requested Stimulus"=w483, "Parameters to Measure"=w482, "Data to Write"=enum16{"Calibration", "Display", "De-Embed"}."Calibration") -> ("error out"=w501:errorcluster)  [unwired: 2 in, 5 out]
                n107 = Select(t="ABORT", s=w501, f=w486) -> (s? t:f=w505:string)
              }
              frame "Abort" {
                n108 = call "SP Clear Calibration From INI File.vi"("error in (no error)"=w569, "Parameters to Measure"=w564) -> ("error out"=w568:errorcluster)  [unwired: 9 out]
              }
              frame "Abort All" {
                n109 = call "SP Clear Calibration From INI File.vi"("error in (no error)"=w577, "Parameters to Measure"=w572) -> ("error out"=w576:errorcluster)  [unwired: 9 out]
              }
            }
          }
        }
      }
    }
  }
  "Next Action" <- w43
  "Parameters to Measure" <- w42
  "Timing Metrics Out" <- w35
  n110 = call "Set LabVIEW VI Topmost.vi"("error in (no error)"=w30, "VI Refnum (null)"="Parent VI Refnum") -> ("error out"=→"error out":errorcluster)  [unwired: 7 in, 2 out]
  n111 = for {
    tunnel: [w584] -> w10 mode=indexing
    tunnel: w42 -> [w583] mode=indexing
    shift-right: [w581] -> w8
    shift-left: w5 -> [w580]
    n112 = Unbundle By Name(w583) -> ("Calibration.String"=w582:string, "Calibration.State"=w584:bool)
    n113 = case shown="Default" w582 {
      selector: w582 -> [w585 _]
      tunnel: [w585 w586] -> w581
      tunnel: w580 -> [_ w586]
      frame Default {
      }
      frame "Not Calibrated" {
      }
    }
  }
  n114 = And Array Elements(Boolean array=w10) -> (logical AND=w6:bool)
  n115 = Select(t=w8, s=w6, f=w5) -> (s? t:f=w7:string)
  n116 = Bundle By Name(cluster=w9, "Stimulus.VNA Stimulus.Calibration.String"=w7, "Stimulus.VNA Stimulus.Calibration.State"=w6) -> (→"Test Parameters Out":T11)
